vi "merge all hydrolysis.vi"(6 "merge_preexisting":bool, 7 "current_starttime":i32, 8 "error in (no error)":errorcluster, 9 "simulation_starttime":i32, 10 "reactor_names":string, 11 "working_dir":string) -> (0 "error out":errorcluster)   [LabVIEW 2019, in "libFileFunctions.lvlib"]
doc: "void merge_all_hydrolysis(const char* working_dir, const char* reactor_names, int simulation_starttime, int current_starttime);"
uses:
  libFileFunctions.lvlib
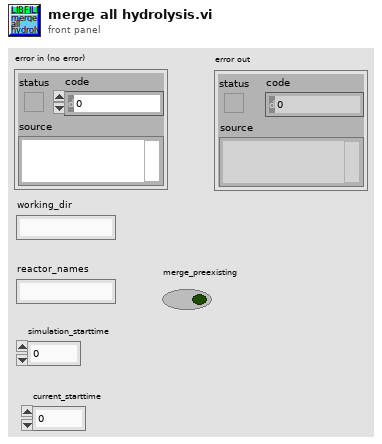
[diagram p1: front panel]
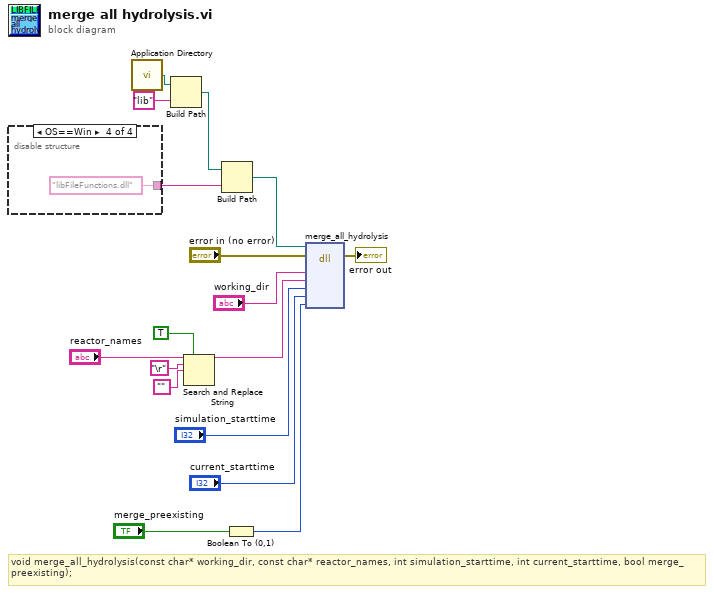
[diagram p0: block diagram]
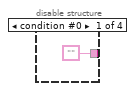
[diagram p2: hidden frame]
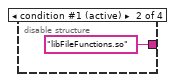
[diagram p3: hidden frame]
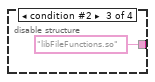
[diagram p4: hidden frame]
diagram:
  # "void merge_all_hydrolysis(const char* working_dir, const char* reactor_names, int simulation_starttime, int current_starttime, bool merge_preexisting);"
  n1 = disable-structure shown="OS==Win" {
    disable-tunnel: ["" "libFileFunctions.so" ("name or relative path") "libFileFunctions.so" ("name or relative path") "libFileFunctions.dll" ("name or relative path")] -> w7
    frame condition #0 {
    }
    frame condition #1 (active) {
    }
    frame condition #2 {
    }
    frame condition #3 {
    }
  }
  n2 = call <vilib>:"Application Directory.vi"() -> ("Application Directory"=w10:path)
  n3 = Build Path(base path=w10, name or relative path="lib") -> (appended path=w8:path)
  n4 = Search and Replace String(replace all?=TRUE ("replace all? (F)"), input string="reactor_names", search string="\r", replace string="") -> (result string=w1:string)  [unwired: 4 in, 3 out]
  n5 = Build Path(base path=w8, name or relative path=w7) -> (appended path=w6:path)
  n6 = Boolean To (0,1)(Boolean="merge_preexisting") -> (0, 1=w11:i16)
  n7 = dll-call lib="home/paul/Schreibtisch/Biogas_plant_setup/LabView/lib/libFileFunctions/libFileFunctions.*" fn="merge_all_hydrolysis"(path in=w6, error in="error in (no error)", "working_dir"="working_dir", "reactor_names"=w1, "simulation_starttime"="simulation_starttime", "current_starttime"="current_starttime", "merge_preexisting"=w11) -> (error out=→"error out":errorcluster)  [unwired: 7 in, 1 out]
